vi "穿管检测信息存储 - NG.vi"(10 "x > y?":bool, 11 "布尔":bool) -> ()   [LabVIEW 2017]
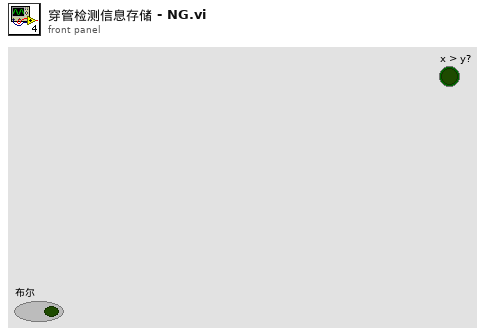
[diagram p1: front panel]
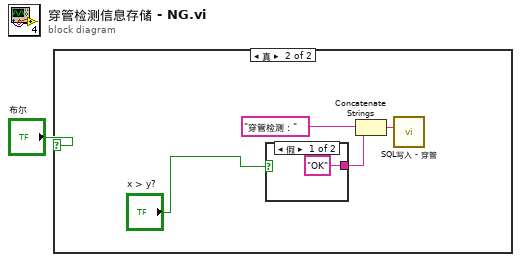
[diagram p0: block diagram]
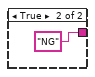
[diagram p3: hidden frame]
diagram:
  n1 = case shown="真" "布尔" {
    frame False {
    }
    frame True {
      n2 = case shown="假" "x > y?" {
        tunnel: ["OK" "NG"] -> w3
        frame False {
        }
        frame True {
        }
      }
      n3 = Concatenate Strings("穿管检测：", w3) -> (w4:string)
      n4 = call "SQL写入 - 穿管.vi"("TestMessage"=w4) -> ()  [unwired: 14 in, 1 out]
    }
  }
